vi "Mpu6050 Read.vi"(4 "error in":errorcluster, 5 "read buffer":string) -> (0 "AccZ":dbl, 1 "error out":errorcluster, 2 "Waveform Chart":cluster{dbl, dbl}(graph))   [LabVIEW 2019]
panel:
  out "Y":dbl
  out "X":dbl
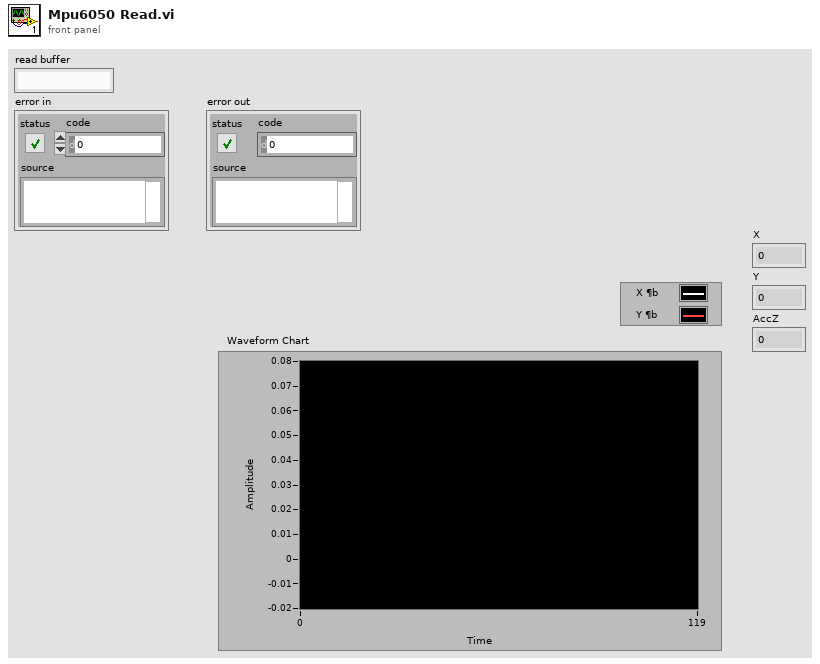
[diagram p1: front panel]
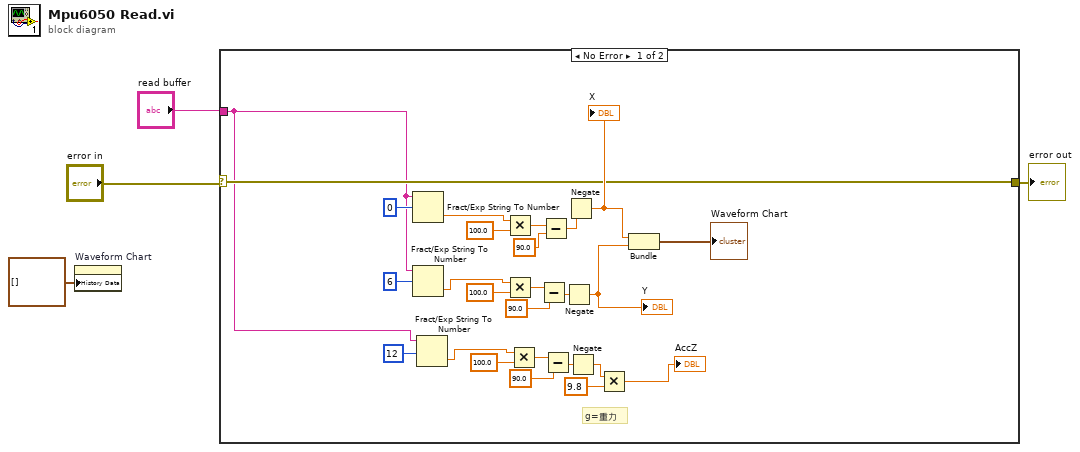
[diagram p0: block diagram]
diagram:
  n1 = property on="Waveform Chart" class="WFChart (strict)"("History Data"=cluster{dbl, dbl}[] []) -> ()  [unwired: 2 in, 2 out]
  n2 = case shown="No Error" "error in" {
    selector: "error in" -> [w17 w31]
    tunnel: [w17 w31] -> w1
    tunnel: "read buffer" -> [w9 _]
    frame No Error {
      # "g=重力"
      n3 = Fract/Exp String To Number(string=w9, offset=0) -> (number=w25:dbl)  [unwired: 2 in, 1 out]
      n4 = Fract/Exp String To Number(string=w9, offset=6) -> (number=w24:dbl)  [unwired: 2 in, 1 out]
      n5 = Fract/Exp String To Number(string=w9, offset=12) -> (number=w13:dbl)  [unwired: 2 in, 1 out]
      n6 = Multiply(x=w25, y=100.0) -> (x*y=w30:dbl)
      n7 = Multiply(x=w24, y=100.0) -> (x*y=w29:dbl)
      n8 = Multiply(x=w13, y=100.0) -> (x*y=w14:dbl)
      n9 = Subtract(x=w29, y=90.0) -> (x-y=w16:dbl)
      n10 = Subtract(x=w30, y=90.0) -> (x-y=w19:dbl)
      n11 = Subtract(x=w14, y=90.0) -> (x-y=w10:dbl)
      n12 = Negate(x=w16) -> (-x=w15:dbl)
      "Y" <- w15
      n13 = Negate(x=w19) -> (-x=w18:dbl)
      "X" <- w18
      n14 = Negate(x=w10) -> (-x=w7:dbl)
      n15 = Multiply(x=w7, y=9.8) -> (x*y=→"AccZ":dbl)
      n16 = Bundle(w18, w15) -> (→"Waveform Chart":cluster{dbl, dbl})  [unwired: 1 in]
    }
    frame Error {
    }
  }
  "error out" <- w1
